vi "Configure RX Port FIFO.vi"(7 "Read Block Size (Samples per Read)":u32, 8 "error in (no error)":errorcluster, 9 "Host Buffer Depth (# of Read Blocks)":u32, 10 "RX Stream Index":i32, 11 "Refnum in":refnum<k20>) -> (0 "error out":errorcluster, 2 "Actual Depth":u32, 3 "Refnum out":refnum<k20>)   [LabVIEW 2023]
uses:
  <vilib>/Utility/error.llb/Error Cluster From Error Code.vi
  <vilib>/rvi/interface/common/niFpgaWaitOnOcc.vi
  <vilib>/rvi/interface/nirviMethod/nirviMethod.xnode
  <vilib>/rvi/errors/niLvFpgaMergeErrorWithErrorCode.vi
  <instrlib>/_niInstr/Streaming/v1/Host/niInstr Streaming v1 Host.lvlib
  <vilib>/FPGAPlugInAG/Dynamic/niLvFpga_StopFifo_Dynamic.vi
  <vilib>/FPGAPlugInAG/Dynamic/niLvFpga_ConfigureFifo_Dynamic.vi
  <vilib>/FPGAPlugInAG/Dynamic/niLvFpga_StartFifo_Dynamic.vi
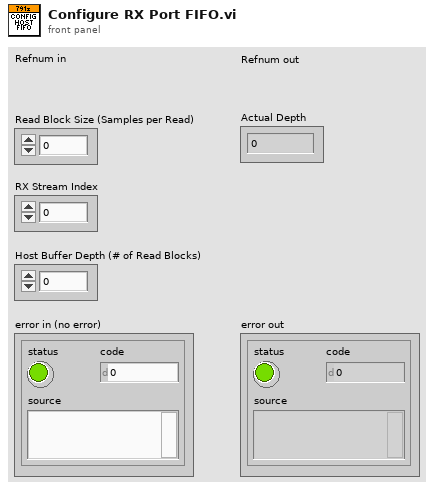
[diagram p1: front panel]
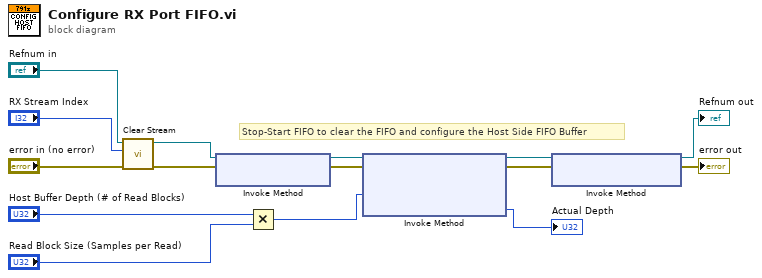
[diagram p0: block diagram]
diagram:
  # "Stop-Start FIFO to clear the FIFO and configure the Host Side FIFO Buffer"
  n1 = call <instrlib>:"Clear Stream.vi"("error in (no error)"="error in (no error)", "stream index"="RX Stream Index", "refnum in"="Refnum in") -> ("error out"=w4:errorcluster, "refnum out"=w11:refnum<k20>)  [unwired: 7 in]
  n2 = xnode "Invoke Method"("FPGA VI Reference In"=w11, "error in"=w4) -> ("FPGA VI Reference Out"=w12:refnum<k20>, "error out"=w10:errorcluster)
  n3 = Multiply(x="Host Buffer Depth (# of Read Blocks)", y="Read Block Size (Samples per Read)") -> (x*y=w6:u32)
  n4 = xnode "Invoke Method"("FPGA VI Reference In"=w12, "error in"=w10, "Requested Depth"=w6) -> ("FPGA VI Reference Out"=w1:refnum<k20>, "error out"=w2:errorcluster, "Actual Depth"=→"Actual Depth":u32)
  n5 = xnode "Invoke Method"("FPGA VI Reference In"=w1, "error in"=w2) -> ("FPGA VI Reference Out"=→"Refnum out":refnum<k20>, "error out"=→"error out":errorcluster)
